vi "Global RefNums.vi"() -> ()   [LabVIEW 2014]
panel:
  in  "Can Smacker":string="Can Smacker"
  in  "Can Grabber Left":string="Can Grabber Left"
  in  "Can Grabber Right":string="Can Grabber Right"
  in  "Sonar Left Side":string="Sonar Left Side"
  in  "IR":string="IR"
  in  "Sonar Right":string="Sonar Right"
  in  "Sonar Left":string="Sonar Left"
  in  "Lift Switch Right":string="Lift Switch Right"
  in  "Fork Sensor":string="Lift Encoder Right"
  in  "Fork Motor":string="Lift Encoder Right"
  in  "Compressor":string="Compressor"
  in  "Lift Switch Left":string="Lift Switch Left"
  in  "Roller Arm Right":string="Roller Arm Right"
  in  "Roller Arm Left":string="Roller Arm Left"
  in  "Roller Right":string="Roller Right"
  in  "Roller Left":string="Roller Left"
  in  "Lift Encoder Right":string="Lift Encoder Right"
  in  "Lift Encoder Left":string="Lift Encoder Left"
  in  "Lift Right":string="Lift Right"
  in  "Lift Left":string="Lift Left"
  in  "Drive Encoder BR":string="Drive Encoder BR"
  in  "Drive Encoder BL":string="Drive Encoder BL"
  in  "Drive Encoder FR":string="Drive Encoder FR"
  in  "Drive Encoder FL":string="Drive Encoder FL"
  in  "NavX":string="NavX"
  in  "Joystick Driver":string="Joystick Driver"
  in  "Joystick Operator":string="Joystick Operator"
  in  "Angle Resolver BR":string="Angle Resolver BR"
  in  "Angle Resolver BL":string="Angle Resolver BL"
  in  "Angle Resolver FR":string="Angle Resolver FR"
  in  "Angle Resolver FL":string="Angle Resolver FL"
  in  "Steer BR":string="Steer BR"
  in  "Steer BL":string="Steer BL"
  in  "Steer FR":string="Steer FR"
  in  "Steer FL":string="Steer FL"
  in  "Drive BR":string="Drive BR"
  in  "Drive BL":string="Drive BL"
  in  "Drive FR":string="Drive FR"
  in  "Drive FL":string="Drive FL"
  # "Actuators"
  # "Sensors"
  # "Fork"
  # "Drive"
  # "Sonar"
  # "Joystick"
  # "Compressor"
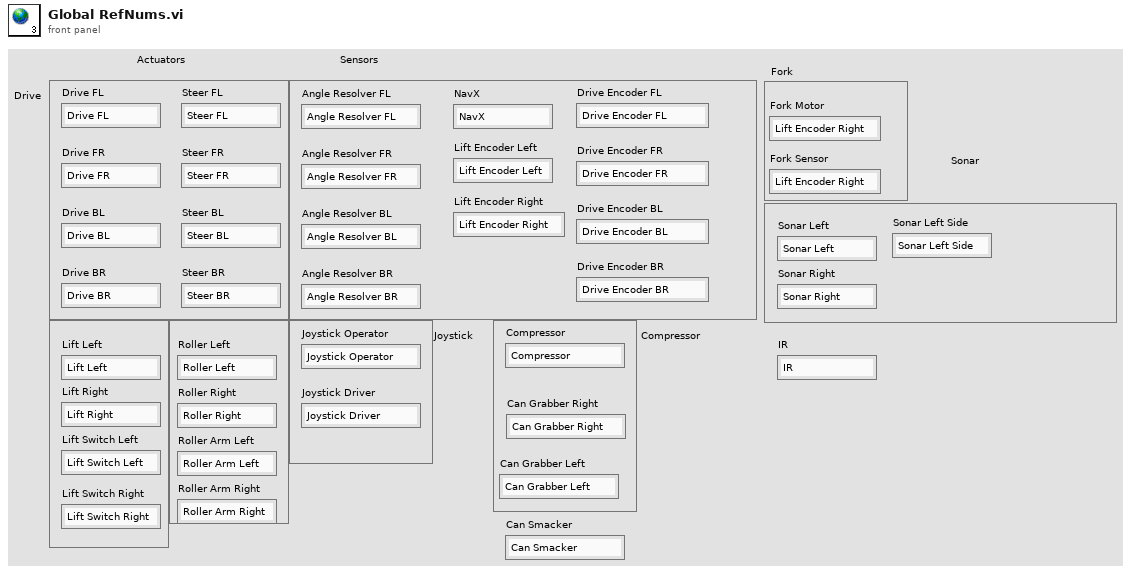
[diagram p1: front panel]
diagram:
